vi "规范时间戳.vi"(11 "字符串":string) -> (3 "result string":string)   [LabVIEW 2016]
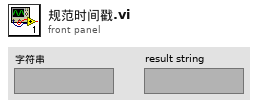
[diagram p1: front panel]
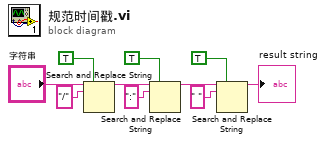
[diagram p0: block diagram]
diagram:
  n1 = Search and Replace String(replace all?=TRUE ("替换全部？(F)"), input string="字符串", search string="/" ("搜索字符串")) -> (result string=w4:string)  [unwired: 5 in, 3 out]
  n2 = Search and Replace String(replace all?=TRUE ("替换全部？(F)"), input string=w4, search string=":" ("搜索字符串")) -> (result string=w8:string)  [unwired: 5 in, 3 out]
  n3 = Search and Replace String(replace all?=TRUE ("替换全部？(F)"), input string=w8, search string=" " ("搜索字符串")) -> (result string=→"result string":string)  [unwired: 5 in, 3 out]
